vi "main.vi"() -> ()   [LabVIEW 2015]
uses:
  controls/state.ctl
  controls/message.ctl
  controls/filestatus.ctl
  controls/users ind.ctl
  controls/user.ctl
  controls/enterstatus.ctl
  controls/nextstate.ctl
panel:
  out "error out":errorcluster
  in  "error in":errorcluster
  in  "Enter":bool
  in  "User Input":string
  in  "Right Buttons":T1
  out "Right Menu":T2
  in  "Left Buttons":T1
  out "Left Menu":T2
  in  "Card Simulator":bool
  out "ATM Messages":string
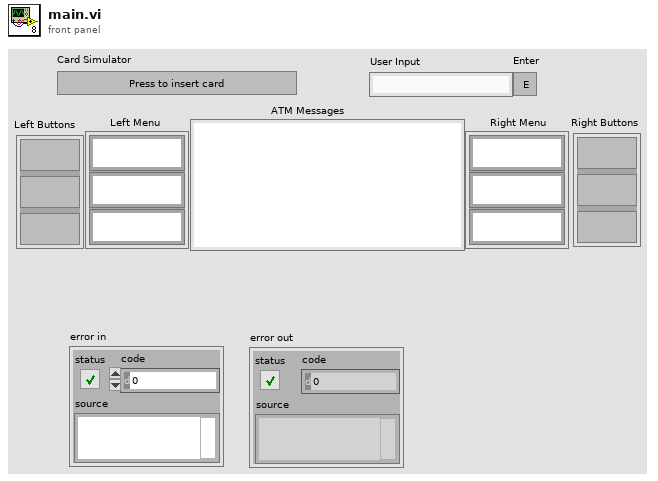
[diagram p1: front panel]
types:
  T1 = cluster{"Func Button":bool, "Func Button 2":bool, "Func Button 3":bool}
  T2 = cluster{"RFS String":string, "RFS String 2":string, "RFS String 3":string}
  T3 = enum8{"Enabled", "Disabled", "Disabled and Grayed Out"}
  T4 = typedef "state.ctl" = enum16{"Shutdown", "Run", "Initialize"}
  T5 = typedef "message.ctl" = enum16{"Deposit Complete", "Welcome", "Menu", "Verification Failed", "Session Terminate", "Deposit", "Withdrawal", "Withdrawal Complete", "Withdrawal Failed", "Balance Inq"}
  T6 = typedef "filestatus.ctl" = enum16{"Write", "Read"}
  T7 = typedef "user.ctl" = cluster{"Code":string, "Full Name":string, "Balance":string}
  T8 = typedef "nextstate.ctl" = enum16{"Fast Cash", "Withdraw", "Deposit", "Validate"}
  T9 = typedef "enterstatus.ctl" = enum16{"Set", "Get"}
  T10 = typedef "users ind.ctl" = cluster{"Users":T7[], "User num":i32}
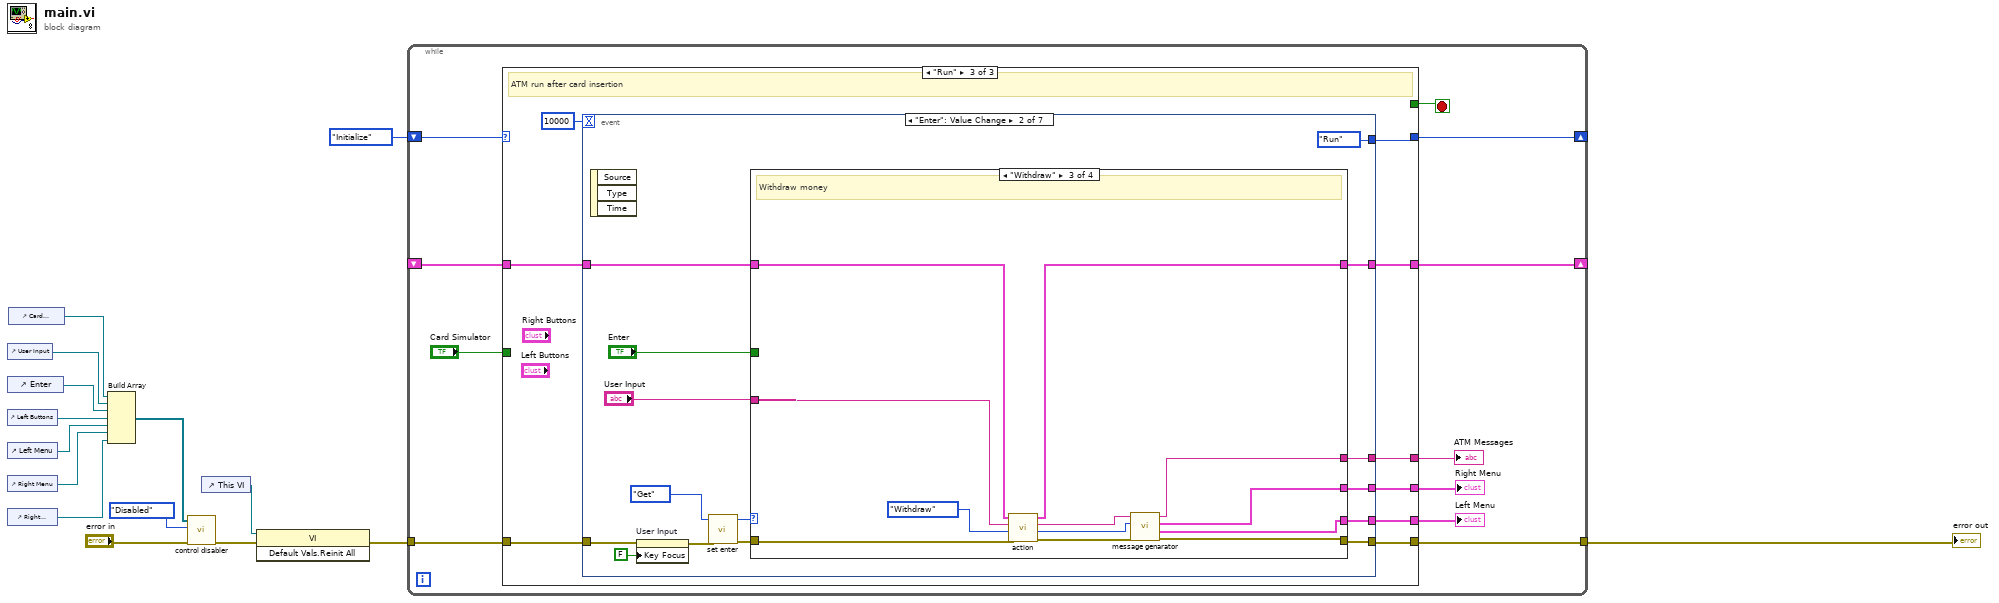
[diagram p0: block diagram]
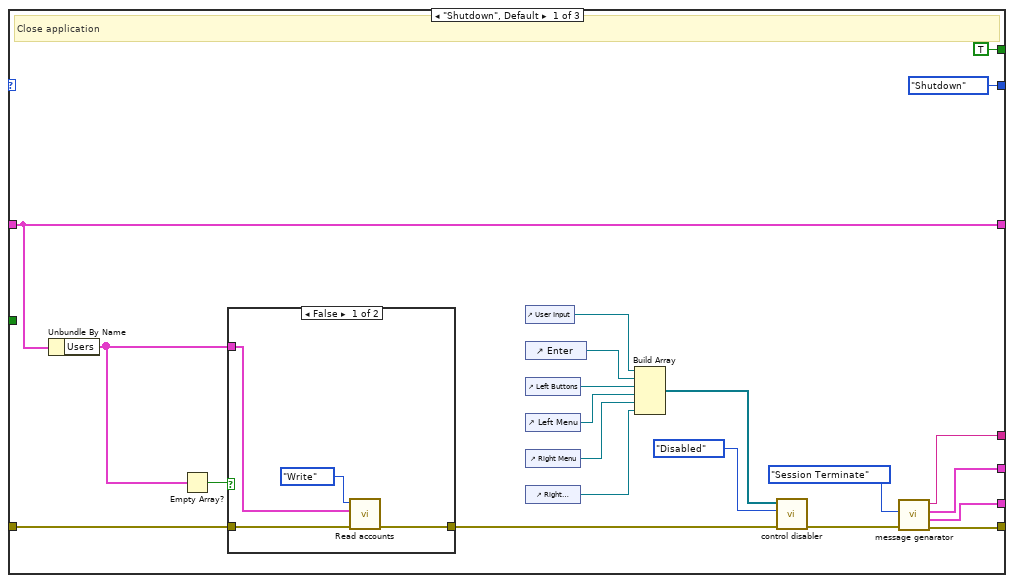
[diagram p2: hidden frame]
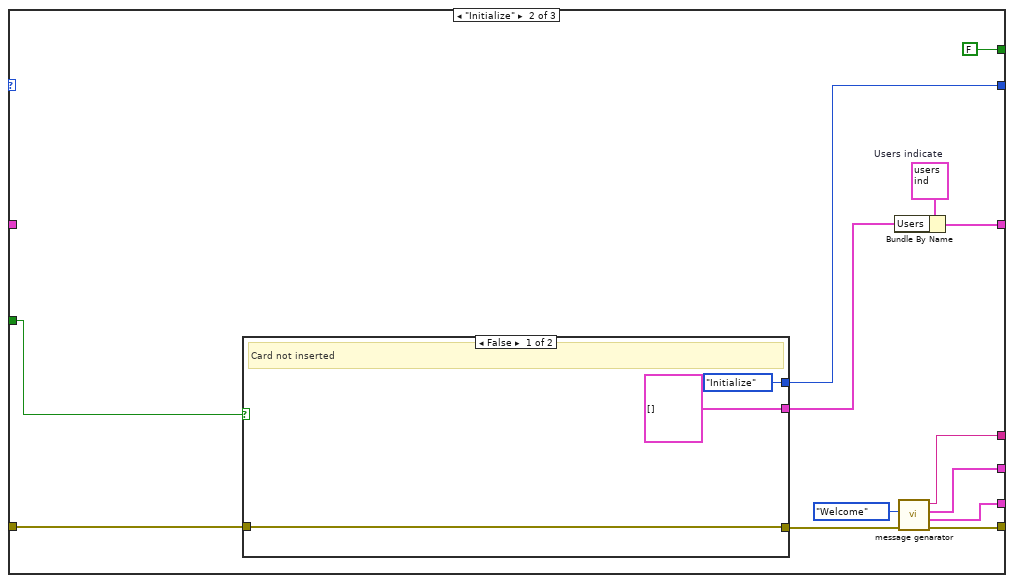
[diagram p4: hidden frame]
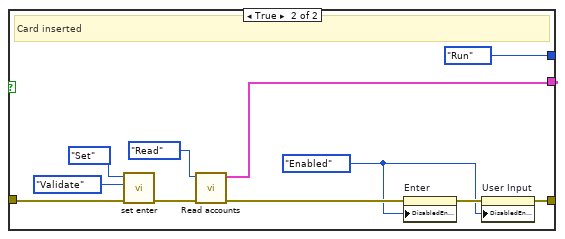
[diagram p5: hidden frame]
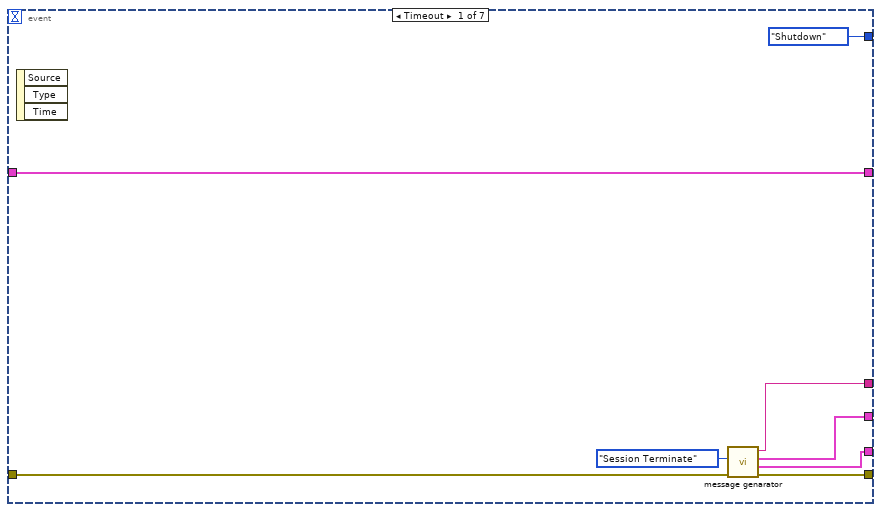
[diagram p6: hidden frame]
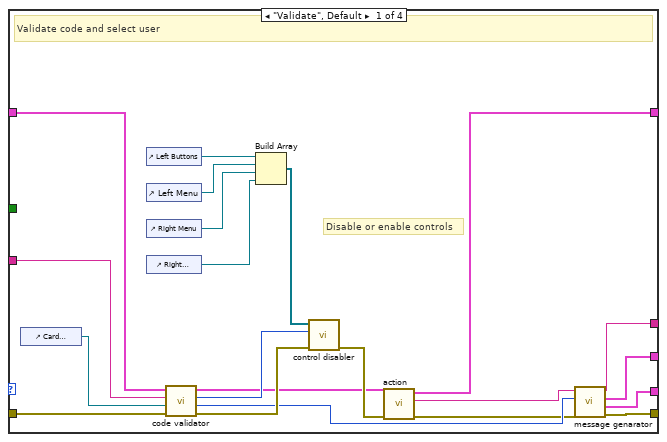
[diagram p7: hidden frame]
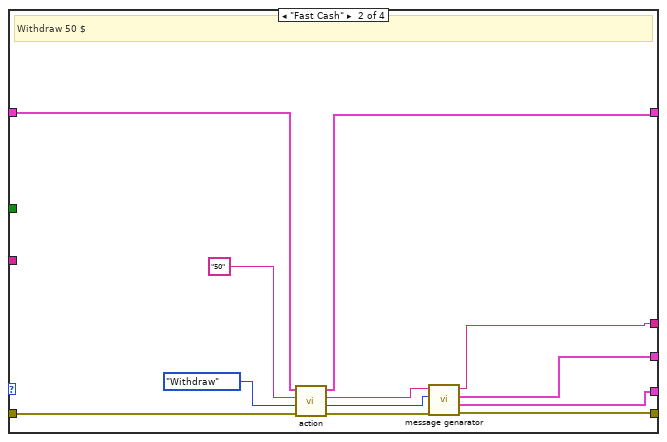
[diagram p8: hidden frame]
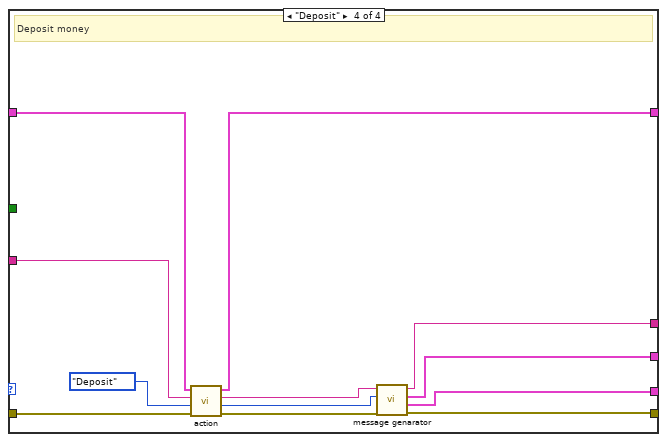
[diagram p9: hidden frame]
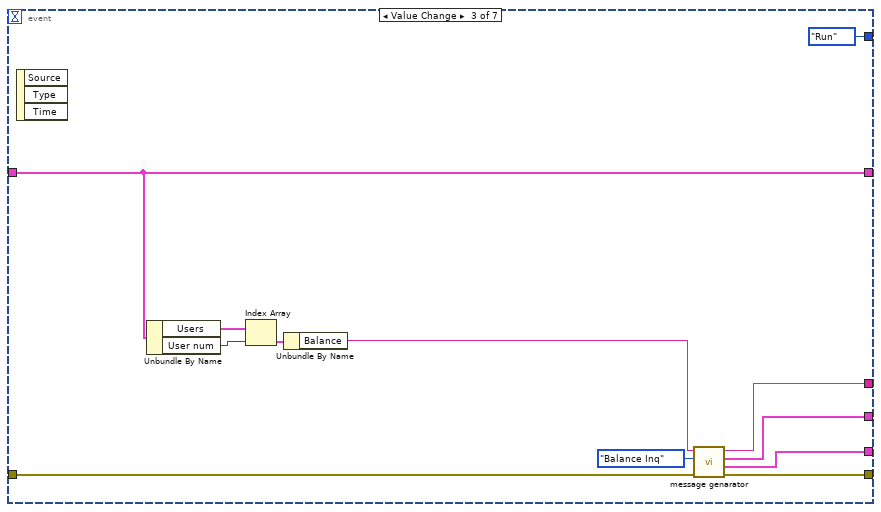
[diagram p10: hidden frame]
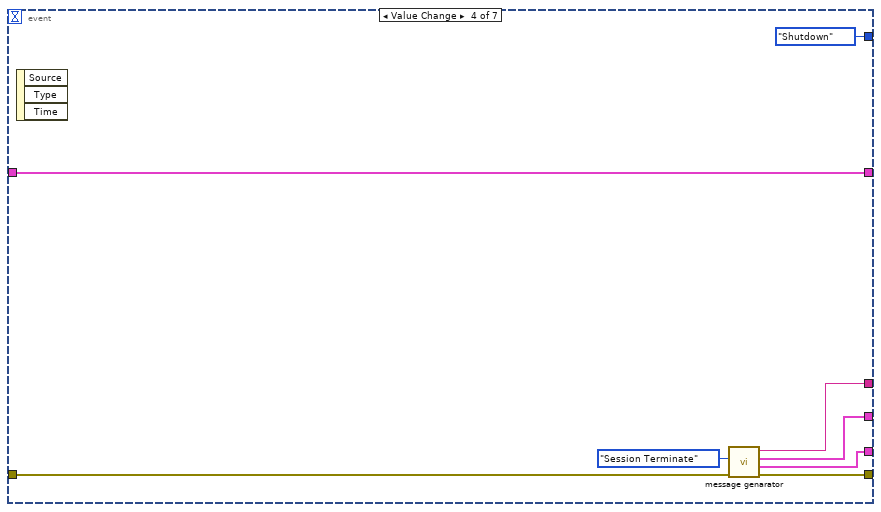
[diagram p11: hidden frame]
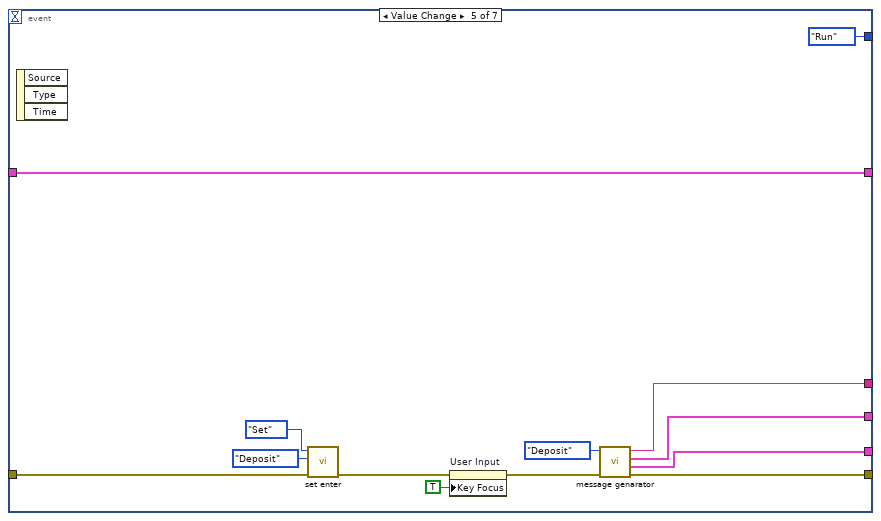
[diagram p12: hidden frame]
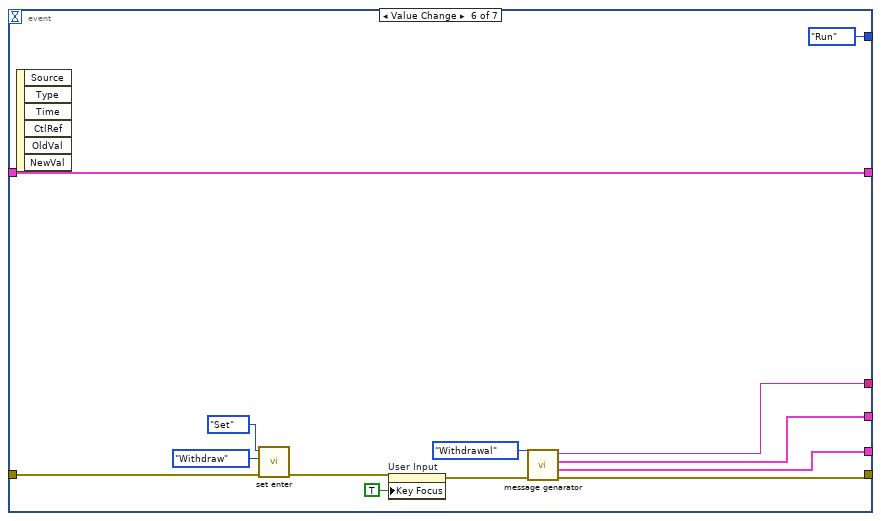
[diagram p13: hidden frame]
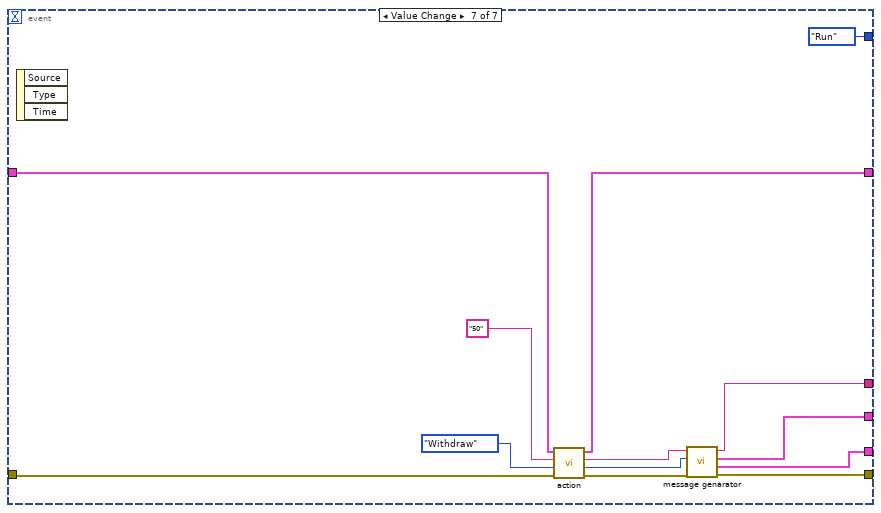
[diagram p14: hidden frame]
diagram:
  n1 = control-ref of="User Input"() -> (w13:refnum<vi>)
  n2 = control-ref of="Enter"() -> (w12:refnum<vi>)
  n3 = control-ref of="Left Buttons"() -> (w11:refnum<vi>)
  n4 = control-ref of="Left Menu"() -> (w10:refnum<vi>)
  n5 = control-ref of="Right Menu"() -> (w9:refnum<vi>)
  n6 = control-ref of="Right Buttons"() -> (w8:refnum<vi>)
  n7 = control-ref of="Card Simulator"() -> (w1:refnum<vi>)
  n8 = Build Array(w1, w13, w12, w11, w10, w9, w8) -> (w7:refnum<vi>[])
  n9 = call "control disabler.vi"("error in (no error)"="error in", "Disabled"=T3."Disabled", "Array"=w7) -> ("error out"=w4:errorcluster)  [unwired: 8 in]
  n10 = control-ref of="This VI"() -> (w2:refnum<vi>)
  n11 = invoke class="VI" method="Default Vals.Reinit All"(reference=w2, error in=w4) -> (error out=w3:errorcluster)  [unwired: 1 in, 2 out]
  n12 = while {
    tunnel: w3 -> [w25]
    tunnel: [w24] -> w14
    shift-right: [w21] -> _
    shift-left: _ -> [w16]
    shift-right: [w17] -> _
    shift-left: state."Initialize" ("state") -> [w26]
    stop <- w22 stop-if-true
    n13 = case shown="\"Run\"" w26 {
      tunnel: w25 -> [w39 w65 w87]
      tunnel: [w31 w58 w83] -> w24
      tunnel: "Card Simulator" -> [_ w64 _]
      tunnel: [TRUE FALSE _] -> w22
      tunnel: [w36 w60 w84] -> w21
      tunnel: [w29 w56 w82] -> w20
      tunnel: [w30 w55 w81] -> w19
      tunnel: [w32 w54 w80] -> w18
      tunnel: [state."Shutdown" ("state") w53 w86] -> w17
      tunnel: w16 -> [w36 _ w85]
      frame "Shutdown", Default {
        # "Close application"
        n14 = Unbundle By Name(w36) -> ("Users"=w35:T7[])
        n15 = Empty Array?(array=w35) -> (empty?=w37:bool)
        n16 = case shown="False" w37 {
          tunnel: w39 -> [w50 w52]
          tunnel: [w49 w52] -> w38
          tunnel: w35 -> [w48 _]
          frame False {
            n17 = call "Read accounts.vi"("error in"=w50, "Users in"=w48, "filestatus"=filestatus."Write") -> ("error out"=w49:errorcluster)  [unwired: 7 in, 1 out]
          }
          frame True {
          }
        }
        n18 = control-ref of="User Input"() -> (w41:refnum<vi>)
        n19 = control-ref of="Enter"() -> (w42:refnum<vi>)
        n20 = control-ref of="Left Buttons"() -> (w43:refnum<vi>)
        n21 = control-ref of="Left Menu"() -> (w44:refnum<vi>)
        n22 = control-ref of="Right Menu"() -> (w45:refnum<vi>)
        n23 = control-ref of="Right Buttons"() -> (w46:refnum<vi>)
        n24 = Build Array(w41, w42, w43, w44, w45, w46) -> (w47:refnum<vi>[])
        n25 = call "control disabler.vi"("error in (no error)"=w38, "Disabled"=T3."Disabled", "Array"=w47) -> ("error out"=w33:errorcluster)  [unwired: 8 in]
        n26 = call "message genarator.vi"("error in"=w33, "Message in"=message."Session Terminate") -> ("error out"=w31:errorcluster, "Left Menu"=w32:T2, "Right Menu"=w30:T2, "Message out"=w29:string)  [unwired: 6 in]
      }
      frame "Initialize" {
        w62 = T10 {"Users"=[{"Code"="12345", "Full Name"="John  Doe", "Balance"="550"}, {"Code"="23456", "Full Name"="Jennifer  Rodriguez", "Balance"="1000"}, {"Code"="34567", "Full Name"="Bryan  Smitch", "Balance"="750"}, {"Code"="45678", "Full Name"="Julie  Ramirez", "Balance"="900"}], "User num"=0}  # Users indicate
        n27 = case shown="False" w64 {
          tunnel: w65 -> [w67 w73]
          tunnel: [w67 w76] -> w59
          tunnel: [T7[] [] ("Users") w74] -> w61
          tunnel: [state."Initialize" ("state") state."Run" ("state")] -> w53
          frame False {
            # "Card not inserted"
          }
          frame True {
            w75 = T3."Enabled" ("Disabled")
            # "Card inserted"
            n28 = call "set enter.vi"("error in"=w73, "nextstate in"=nextstate."Validate", "enterstate"=enterstatus."Set") -> ("error out"=w72:errorcluster)  [unwired: 7 in, 1 out]
            n29 = call "Read accounts.vi"("error in"=w72, "filestatus"=filestatus."Read") -> ("error out"=w78:errorcluster, "Users"=w74:T7[])  [unwired: 8 in]
            n30 = property on="Enter" class="Bool"(error in=w78, "DisabledEnum"=w75) -> (error out=w77:errorcluster)  [unwired: 1 in, 1 out]
            n31 = property on="User Input" class="Str"(error in=w77, "DisabledEnum"=w75) -> (error out=w76:errorcluster)  [unwired: 1 in, 1 out]
          }
        }
        n32 = Bundle By Name(cluster=w62, "Users"=w61) -> (w60:T10)
        n33 = call "message genarator.vi"("error in"=w59, "Message in"=message."Welcome") -> ("error out"=w58:errorcluster, "Left Menu"=w54:T2, "Right Menu"=w55:T2, "Message out"=w56:string)  [unwired: 6 in]
      }
      frame "Run" {
        # "ATM run after card insertion"
        n34 = event shown="[1] \"Enter\": Value Change" {
          selector: _ -> [_ _ _ _ _ _ _]
          dyn-events: _ -> [_ _ _ _ _ _ _]
          timeout: 10000 -> [_ _ _ _ _ _ _]
          tunnel: w87 -> [w93 w101 w177 w188 w201 w214 w221]
          tunnel: [state."Shutdown" ("state") state."Run" ("state") state."Run" ("state") state."Shutdown" ("state") state."Run" ("state") state."Run" ("state") state."Run" ("state")] -> w86
          tunnel: w85 -> [w95 w108 w170 w182 w190 w203 w216]
          tunnel: [w95 w102 w170 w182 w190 w203 w215] -> w84
          tunnel: [w92 w107 w174 w187 w194 w208 w220] -> w83
          tunnel: [w91 w104 w171 w183 w191 w205 w217] -> w82
          tunnel: [w90 w105 w172 w184 w192 w206 w218] -> w81
          tunnel: [w89 w106 w173 w185 w193 w207 w219] -> w80
          event Timeout {
            n35 = event-data() -> ()  [unwired: 1 in, 3 out]
            n36 = call "message genarator.vi"("error in"=w93, "Message in"=message."Session Terminate") -> ("error out"=w92:errorcluster, "Left Menu"=w89:T2, "Right Menu"=w90:T2, "Message out"=w91:string)  [unwired: 6 in]
          }
          event "Enter": Value Change {
            n37 = event-data() -> ()  [unwired: 1 in, 3 out]
            n38 = property on="User Input" class="Str"(error in=w101, "Key Focus"=FALSE) -> (error out=w100:errorcluster)  [unwired: 1 in, 1 out]
            n39 = call "set enter.vi"("error in"=w100, "enterstate"=enterstatus."Get") -> ("error out"=w110:errorcluster, "nextstate out"=w111:T8)  [unwired: 8 in]
            n40 = case shown="\"Withdraw\"" w111 {
              tunnel: w110 -> [w132 w140 w152 w168]
              tunnel: "User Input" -> [w113 _ w151 w167]
              tunnel: w108 -> [w112 w136 w150 w166]
              tunnel: [w123 w139 w149 w164] -> w107
              tunnel: [w122 w138 w145 w160] -> w106
              tunnel: [w121 w134 w146 w159] -> w105
              tunnel: [w120 w133 w147 w158] -> w104
              tunnel: [w116 w135 w148 w161] -> w102
              tunnel: "Enter" -> [_ _ _ _]
              frame "Validate", Default {
                # "Disable or enable controls"
                # "Validate code and select user"
                n41 = control-ref of="Card Simulator"() -> (w114:refnum<vi>)
                n42 = control-ref of="Left Buttons"() -> (w131:refnum<vi>)
                n43 = control-ref of="Left Menu"() -> (w130:refnum<vi>)
                n44 = control-ref of="Right Menu"() -> (w129:refnum<vi>)
                n45 = control-ref of="Right Buttons"() -> (w128:refnum<vi>)
                n46 = call "code validator.vi"("error in"=w132, "Card"=w114, "User Input"=w113, "Users indicate"=w112) -> ("error out"=w126:errorcluster, "Message"=w124:T5, "Buttons"=w125:T3, "Users indicate"=w118:T10)  [unwired: 4 in]
                n47 = Build Array(w131, w130, w129, w128) -> (w127:refnum<vi>[])
                n48 = call "control disabler.vi"("error in (no error)"=w126, "Disabled"=w125, "Array"=w127) -> ("error out"=w119:errorcluster)  [unwired: 8 in]
                n49 = call "action.vi"("error in"=w119, "Users indicate"=w118) -> ("error out"=w115:errorcluster, "Result"=w117:string, "Users indicate  2"=w116:T10)  [unwired: 6 in, 1 out]
                n50 = call "message genarator.vi"("error in"=w115, "Message in"=w124, "Input data"=w117) -> ("error out"=w123:errorcluster, "Left Menu"=w122:T2, "Right Menu"=w121:T2, "Message out"=w120:string)  [unwired: 5 in]
              }
              frame "Fast Cash" {
                # "Withdraw 50 $"
                n51 = call "action.vi"("error in"=w140, "status"=nextstate."Withdraw", "Input"="50" ("User Input"), "Users indicate"=w136) -> ("error out"=w141:errorcluster, "Message"=w143:T5, "Result"=w142:string, "Users indicate  2"=w135:T10)  [unwired: 4 in]
                n52 = call "message genarator.vi"("error in"=w141, "Message in"=w143, "Input data"=w142) -> ("error out"=w139:errorcluster, "Left Menu"=w138:T2, "Right Menu"=w134:T2, "Message out"=w133:string)  [unwired: 5 in]
              }
              frame "Withdraw" {
                # "Withdraw money"
                n53 = call "action.vi"("error in"=w152, "status"=nextstate."Withdraw", "Input"=w151, "Users indicate"=w150) -> ("error out"=w156:errorcluster, "Message"=w154:T5, "Result"=w155:string, "Users indicate  2"=w148:T10)  [unwired: 4 in]
                n54 = call "message genarator.vi"("error in"=w156, "Message in"=w154, "Input data"=w155) -> ("error out"=w149:errorcluster, "Left Menu"=w145:T2, "Right Menu"=w146:T2, "Message out"=w147:string)  [unwired: 5 in]
              }
              frame "Deposit" {
                # "Deposit money"
                n55 = call "action.vi"("error in"=w168, "status"=nextstate."Deposit", "Input"=w167, "Users indicate"=w166) -> ("error out"=w165:errorcluster, "Message"=w162:T5, "Result"=w163:string, "Users indicate  2"=w161:T10)  [unwired: 4 in]
                n56 = call "message genarator.vi"("error in"=w165, "Message in"=w162, "Input data"=w163) -> ("error out"=w164:errorcluster, "Left Menu"=w160:T2, "Right Menu"=w159:T2, "Message out"=w158:string)  [unwired: 5 in]
              }
            }
          }
          event "Left Buttons.Func Button 2": Value Change {
            n57 = event-data() -> ()  [unwired: 1 in, 3 out]
            n58 = Unbundle By Name(w170) -> ("Users"=w180:T7[], "User num"=w179:i32)
            n59 = Index Array(array=w180, index=w179) -> (element=w178:T7)
            n60 = Unbundle By Name(w178) -> ("Balance"=w176:string)
            n61 = call "message genarator.vi"("error in"=w177, "Message in"=message."Balance Inq", "Input data"=w176) -> ("error out"=w174:errorcluster, "Left Menu"=w173:T2, "Right Menu"=w172:T2, "Message out"=w171:string)  [unwired: 5 in]
          }
          event "Left Buttons.Func Button 3": Value Change {
            n62 = event-data() -> ()  [unwired: 1 in, 3 out]
            n63 = call "message genarator.vi"("error in"=w188, "Message in"=message."Session Terminate") -> ("error out"=w187:errorcluster, "Left Menu"=w185:T2, "Right Menu"=w184:T2, "Message out"=w183:string)  [unwired: 6 in]
          }
          event "Right Buttons.Func Button": Value Change {
            n64 = event-data() -> ()  [unwired: 1 in, 3 out]
            n65 = call "set enter.vi"("error in"=w201, "nextstate in"=nextstate."Deposit", "enterstate"=enterstatus."Set") -> ("error out"=w200:errorcluster)  [unwired: 7 in, 1 out]
            n66 = property on="User Input" class="Str"(error in=w200, "Key Focus"=TRUE) -> (error out=w196:errorcluster)  [unwired: 1 in, 1 out]
            n67 = call "message genarator.vi"("error in"=w196, "Message in"=message."Deposit") -> ("error out"=w194:errorcluster, "Left Menu"=w193:T2, "Right Menu"=w192:T2, "Message out"=w191:string)  [unwired: 6 in]
          }
          event "Right Buttons.Func Button 2": Value Change {
            n68 = event-data() -> ()  [unwired: 1 in, 6 out]
            n69 = call "set enter.vi"("error in"=w214, "nextstate in"=nextstate."Withdraw", "enterstate"=enterstatus."Set") -> ("error out"=w211:errorcluster)  [unwired: 7 in, 1 out]
            n70 = property on="User Input" class="Str"(error in=w211, "Key Focus"=TRUE) -> (error out=w209:errorcluster)  [unwired: 1 in, 1 out]
            n71 = call "message genarator.vi"("error in"=w209, "Message in"=message."Withdrawal") -> ("error out"=w208:errorcluster, "Left Menu"=w207:T2, "Right Menu"=w206:T2, "Message out"=w205:string)  [unwired: 6 in]
          }
          event "Right Buttons.Func Button 3": Value Change {
            n72 = event-data() -> ()  [unwired: 1 in, 3 out]
            n73 = call "action.vi"("error in"=w221, "status"=nextstate."Withdraw", "Input"="50" ("User Input"), "Users indicate"=w216) -> ("error out"=w223:errorcluster, "Message"=w225:T5, "Result"=w224:string, "Users indicate  2"=w215:T10)  [unwired: 4 in]
            n74 = call "message genarator.vi"("error in"=w223, "Message in"=w225, "Input data"=w224) -> ("error out"=w220:errorcluster, "Left Menu"=w219:T2, "Right Menu"=w218:T2, "Message out"=w217:string)  [unwired: 5 in]
          }
        }
      }
    }
    "ATM Messages" <- w20
    "Left Menu" <- w18
    "Right Menu" <- w19
  }
  "error out" <- w14
